vi "HEWH Display Draw Message.vi"(11 "Start Draw":dbl) -> (3 "concatenated string":string)   [LabVIEW 2019]
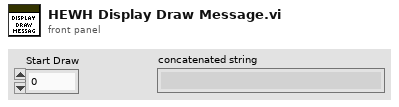
[diagram p1: front panel]
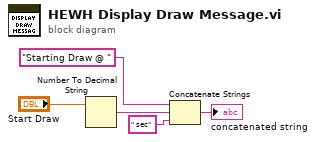
[diagram p0: block diagram]
diagram:
  n1 = Number To Decimal String(number="Start Draw") -> (decimal integer string=w3:string)  [unwired: 1 in]
  n2 = Concatenate Strings("Starting Draw @ " ("string"), w3, " sec" ("string")) -> (→"concatenated string":string)
